vi "Configure Frequency Offset.vi"(6 "LO Frequency (3E9 Hz)":dbl=3000000000.0 format="%^#_9g", 7 "Conversion Mode (0: RF = n * LO + IF)":u16(ring) items=["RF = n * LO + IF", "RF = n * LO - IF"], 8 "error in (no error)":errorcluster, 9 "Frequency Offset Factor (1)":i32=1, 10 "Enable Frequency Offset (Disable)":bool, 11 "VISA resource name":refnum<visa-resource-name>) -> (0 "error out":errorcluster, 3 "VISA resource name out":refnum<visa-resource-name>)   [LabVIEW 2011, in "Agilent E5052X.lvlib"]
doc: "Sets frequency offset settings for the instrument."
uses:
  Agilent E5052X.lvlib
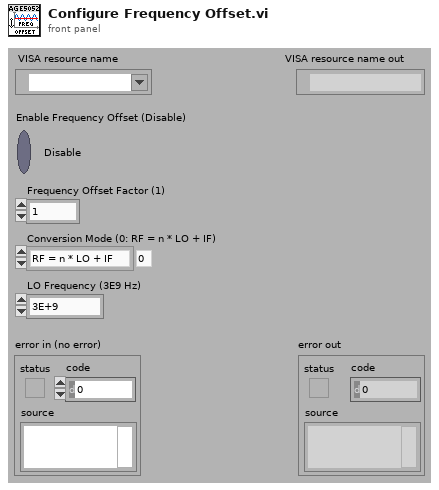
[diagram p1: front panel]
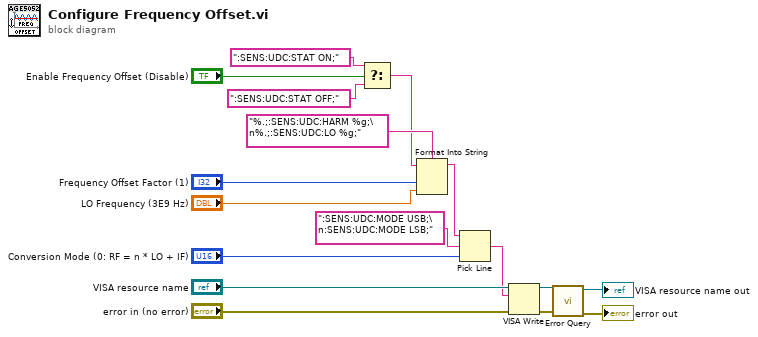
[diagram p0: block diagram]
diagram:
  n1 = Select(t=":SENS:UDC:STAT ON;", s="Enable Frequency Offset (Disable)", f=":SENS:UDC:STAT OFF;") -> (s? t:f=w5:string)
  n2 = Format Into String(format string="%.;:SENS:UDC:HARM %g;\n%.;:SENS:UDC:LO %g;", initial string=w5, "Frequency Offset Factor (1)", "LO Frequency (3E9 Hz)") -> (resulting string=w2:string)  [unwired: 1 in, 1 out]
  n3 = Pick Line(string ("")=w2, multi-line string=":SENS:UDC:MODE USB;\n:SENS:UDC:MODE LSB;", line index="Conversion Mode (0: RF = n * LO + IF)") -> (output string=w1:string)
  n4 = VISA Write(VISA resource name="VISA resource name", write buffer=w1, error in (no error)="error in (no error)") -> (VISA resource name out=w13:refnum<visa-resource-name>, error out=w14:errorcluster)  [unwired: 1 out]
  n5 = call "Error Query.vi"("error in (no error)"=w14, "VISA resource name"=w13) -> ("error out"=→"error out":errorcluster, "VISA resource name out"=→"VISA resource name out":refnum<visa-resource-name>)  [unwired: 6 in, 2 out]
